vi "Get Register.vi"(8 "error in (no error)":errorcluster, 10 "Register Name":string, 11 "Camera in":refnum<class "Camera.lvclass">) -> (0 "error out":errorcluster, 2 "Bytes Out":string, 3 "Camera":refnum<class "Camera.lvclass">)   [LabVIEW 2020, in "Camera.lvclass"]
uses:
  Camera.lvclass
  Camera.lvclass/Camera.ctl
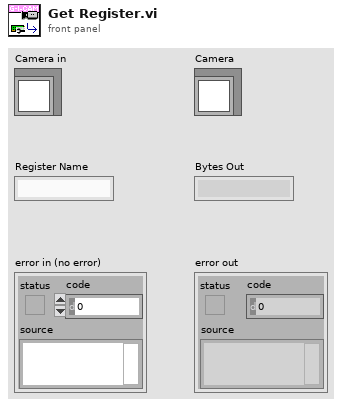
[diagram p1: front panel]
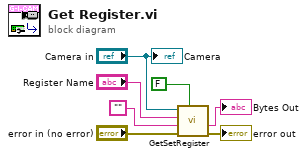
[diagram p0: block diagram]
diagram:
  n1 = call "GetSetRegister.vi"("Set?"=FALSE, "error in (no error)"="error in (no error)", "Bytes in"="", "Register Name"="Register Name", "Camera in"="Camera in") -> ("error out"=→"error out":errorcluster, "Bytes out"=→"Bytes Out":string)  [unwired: 5 in]
  "Camera" <- "Camera in"
